vi "GetAllChanGrpNames.vi"(8 "error in":errorcluster, 11 "TimingGrp in":refnum<class "TimingGrp.lvclass">) -> (0 "error out":errorcluster, 2 "All ChanGrp Names":string[](array[string]))   [LabVIEW 2012, in "Configuration Grandmaster.lvlib" / "TimingGrp.lvclass"]
uses:
  TimingGrp.lvclass
  TimingGrp.lvclass/TimingGrp.ctl
  Class Chan Group/Read GrpName.vi
  Class Chan Group/ChanGrp.lvclass
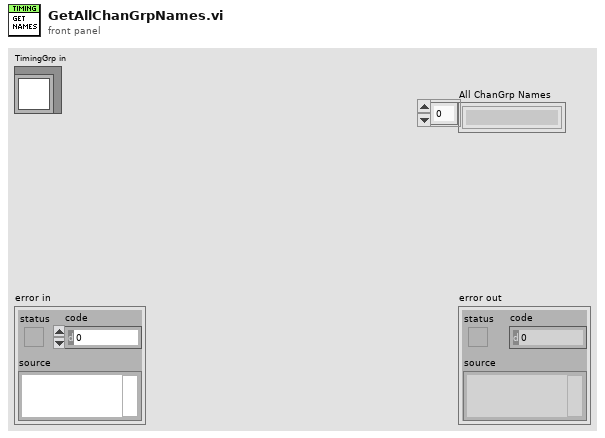
[diagram p1: front panel]
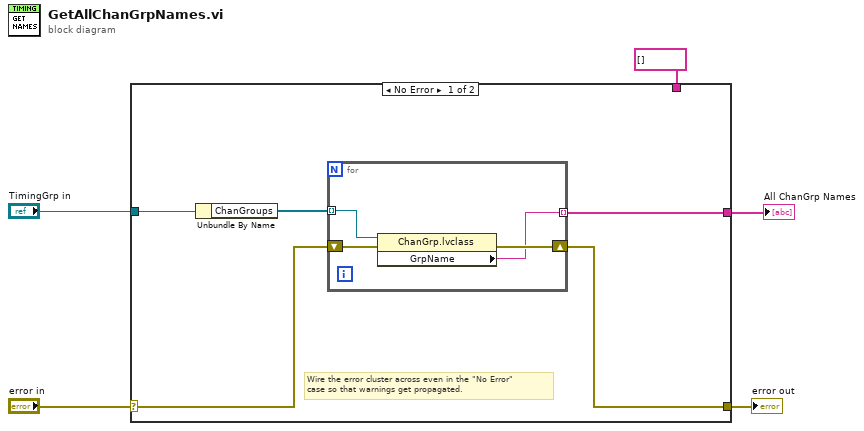
[diagram p0: block diagram]
diagram:
  n1 = case shown="No Error" "error in" {
    selector: "error in" -> [w8 w16]
    tunnel: [w7 w16] -> w4
    tunnel: "TimingGrp in" -> [w10 _]
    tunnel: [w6 w15] -> w2
    tunnel: string[] [] -> [_ w15]
    frame No Error {
      # "Wire the error cluster across even in the \"No Error\"\ncase so that warnings get propagated."
      n2 = Unbundle By Name(w10) -> ("ChanGroups"=w9:refnum<class "ChanGrp.lvclass">[])
      n3 = for {
        tunnel: w9 -> [w14] mode=indexing
        shift-right: [w12] -> w7
        shift-left: w8 -> [w13]
        tunnel: [w11] -> w6 mode=indexing
        n4 = property class="ChanGrp.lvclass"(reference=w14, error in=w13) -> (error out=w12:errorcluster, "GrpName"=w11:string)  [unwired: 1 out]
      }
    }
    frame Error {
    }
  }
  "error out" <- w4
  "All ChanGrp Names" <- w2
